vi "Validate Report Reference.vi"(0 "Report Ref In":T1) -> (1 "Report Ref Out":T1, 2 "Valid":bool)   [LabVIEW 2026, in "XCel Report Engine.lvlib"]
uses:
  XCel Report Engine.lvlib
  Controls/Report Ref.ctl
  C:/Users/m.santucci/Documents/ChatGPT/LV_REPORT_ENGINE/LV/DotNet/XCelReportEngine.dll
  DotNet/XCelReportEngine.dll
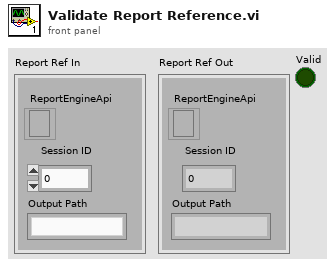
[diagram p1: front panel]
types:
  T1 = typedef "XCel Report Engine.lvlib/Report Ref.ctl" = cluster{"Session ID":i32, "Output Path":string, "ReportEngineApi":refnum<k24>}
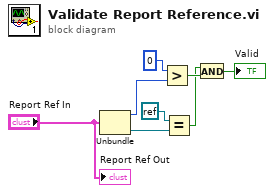
[diagram p0: block diagram]
diagram:
  n1 = Unbundle("Report Ref In") -> ("Session ID"=w5:i32, "ReportEngineApi"=w7:refnum<k24>)  [unwired: 1 out]
  n2 = Greater?(x=0, y=w5) -> (0:w3:bool)
  n3 = Equal?(x=refnum<k0> refnum, y=w7) -> (x = y?=w2:bool)
  n4 = And(x=w2, y=w3) -> (x .and. y?=→"Valid":bool)
  "Report Ref Out" <- "Report Ref In"
